vi "SDSU_ExtractInfo.vi"(8 "error in (no error)":errorcluster, 11 "refnum":i32) -> (0 "error out":errorcluster, 1 "ControllerConfigCluster":T1, 2 "Detector Type":string, 3 "refnum out":i32, 9 "PCI Info":u32[](array[numeric]) format="%.0x", 10 "Config Word Read":u32 format="%.0x")   [LabVIEW 2016]
uses:
  SDSU_GBLVariables.vi
panel:
  in  "get pci info?":bool
  in  "Default type is no info":string="optical"
  in  "Constants":i32(listbox)=5
  in  "Masks":i32(listbox)
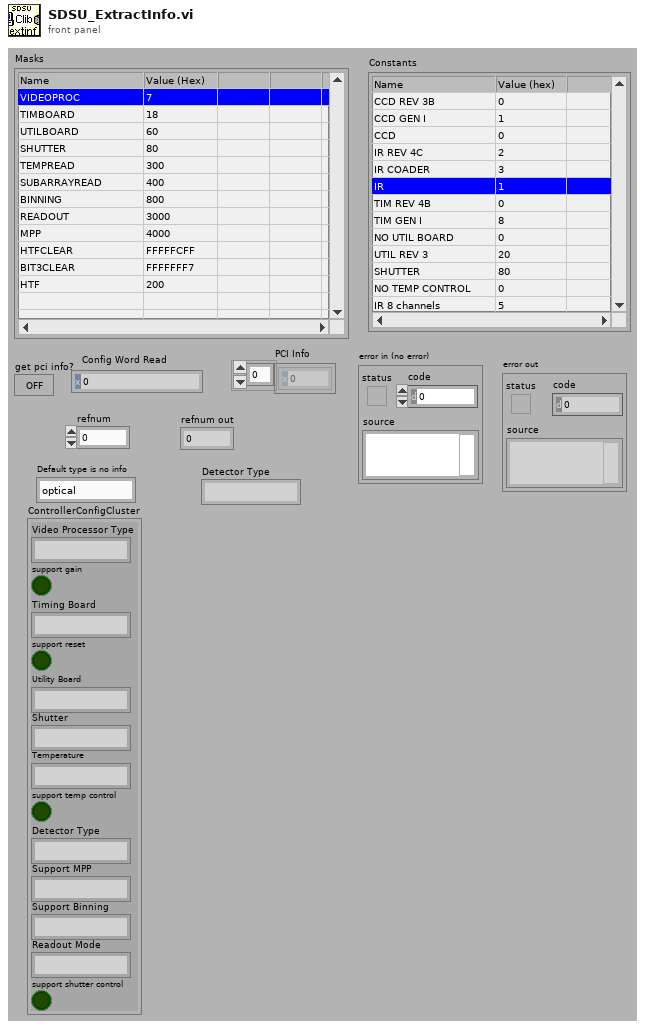
[diagram p1: front panel]
types:
  T1 = cluster{"Video Processor Type":string, "support gain":bool, "Timing Board":string, "support reset":bool, "Utility Board":string, "Shutter":string, "Temperature":string, "support temp control":bool, "Detector Type":string, "Support MPP":string, "Support Binning":string, "Readout Mode":string, "support shutter control":bool}
  T2 = cluster{"VendorID":u32, "DeviceID":u32, "RevisionNumber":u32}
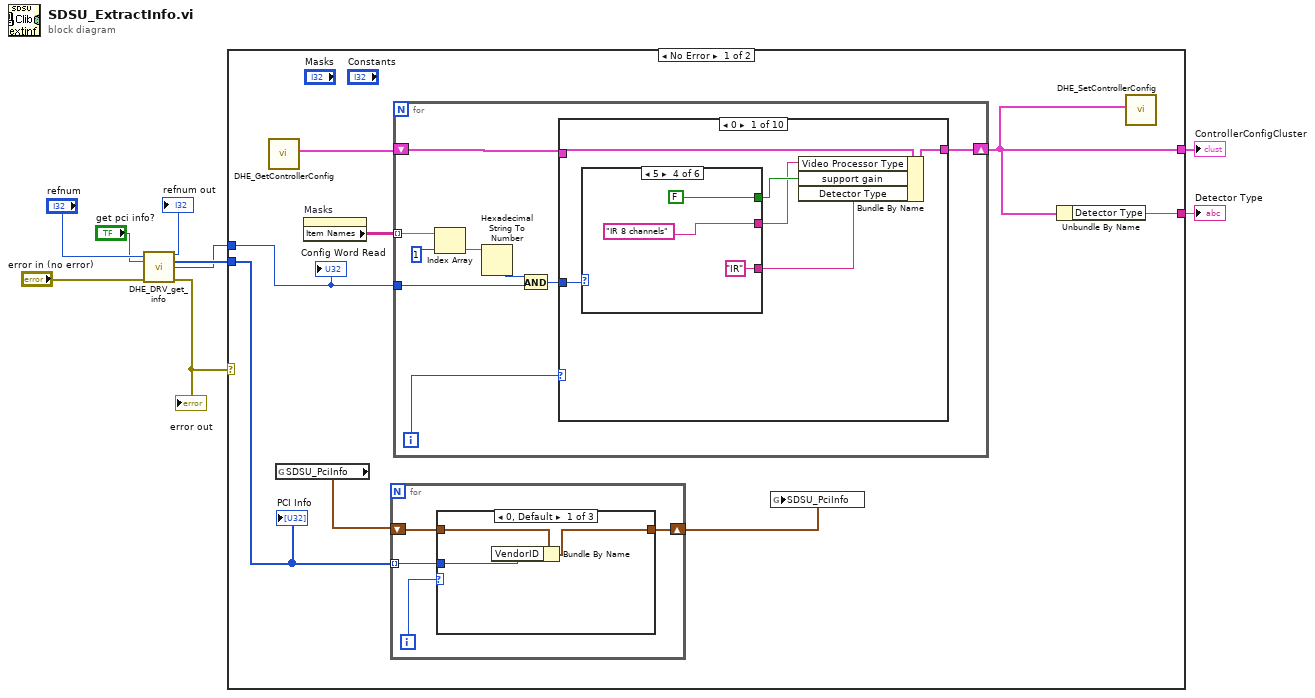
[diagram p0: block diagram]
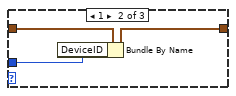
[diagram p2: hidden frame]
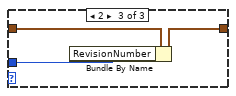
[diagram p3: hidden frame]
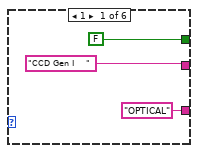
[diagram p4: hidden frame]
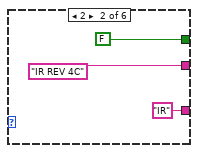
[diagram p5: hidden frame]
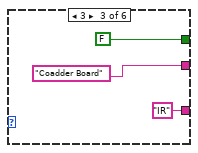
[diagram p6: hidden frame]
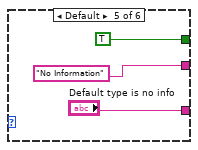
[diagram p7: hidden frame]
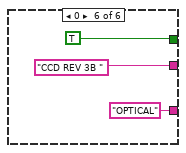
[diagram p8: hidden frame]
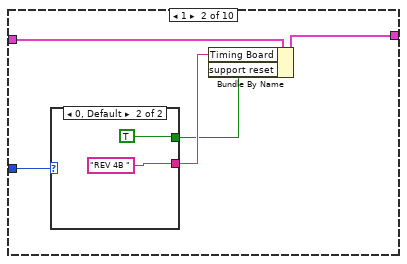
[diagram p9: hidden frame]
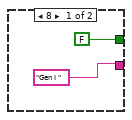
[diagram p10: hidden frame]
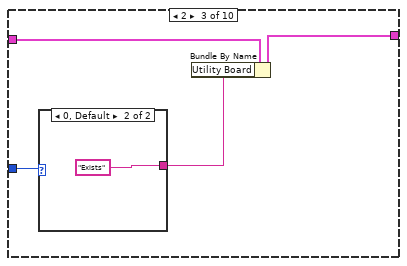
[diagram p11: hidden frame]
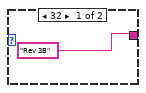
[diagram p12: hidden frame]
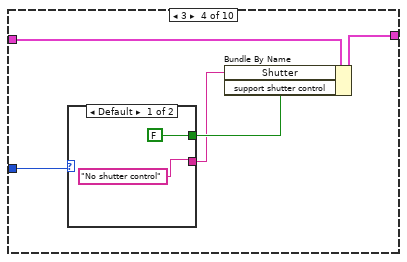
[diagram p13: hidden frame]
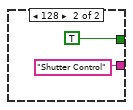
[diagram p14: hidden frame]
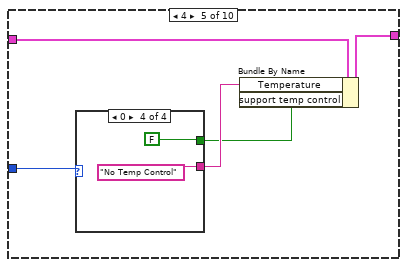
[diagram p15: hidden frame]
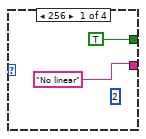
[diagram p16: hidden frame]
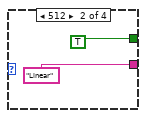
[diagram p17: hidden frame]
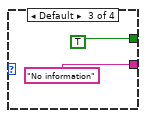
[diagram p18: hidden frame]
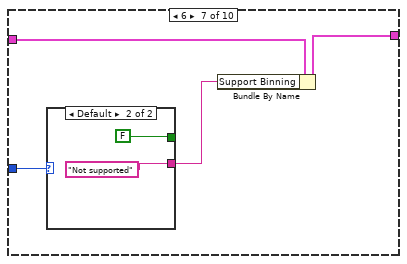
[diagram p20: hidden frame]
diagram:
  n1 = call "DHE_DRV_get_info.vi"("fd"="refnum", "get pci info?"="get pci info?", "error in (no error)"="error in (no error)") -> ("fd"=→"refnum out":i32, "Info"=w8:u16[], "error_code"=w3:i32, "error out"=w9:errorcluster)  [unwired: 9 out]
  "error out" <- w9
  n2 = case shown="No Error" w9 {
    tunnel: w3 -> [w16 _]
    tunnel: w8 -> [w15 _]
    tunnel: [w14 "UNKNOWN" ("Detector Type")] -> w6
    tunnel: [w12 T1 {"Video Processor Type"="", "support gain"=FALSE, "Timing Board"="", "support reset"=FALSE, "Utility Board"="", "Shutter"="", "Temperature"="", "support temp control"=FALSE, "Detector Type"="", "Support MPP"="", "Support Binning"="", "Readout Mode"="", "support shutter control"=FALSE} ("ControllerConfigCluster")] -> w1
    frame No Error {
      n3 = call "DHE_GetControllerConfig.vi"() -> ("ControllerConfigCluster"=w13:T1)  [unwired: 11 out]
      n4 = global read "SDSU_GBLVariables.vi" "SDSU_PciInfo"() -> (w10:T2)
      n5 = property on="Masks" class="MCListbox (strict)"() -> ("Item Names"=w17:string[][])  [unwired: 2 in, 2 out]
      n6 = for {
        tunnel: w15 -> [w19] mode=indexing
        shift-right: [w18] -> w11
        shift-left: w10 -> [w20]
        i -> [w21]
        n7 = case shown="0, Default" w21 {
          tunnel: w20 -> [w24 w27 w30]
          tunnel: w19 -> [w23 w25 w28]
          tunnel: [w22 w26 w29] -> w18
          frame 0, Default {
            n8 = Bundle By Name(cluster=w24, "VendorID"=w23) -> (w22:T2)
          }
          frame 1 {
            n9 = Bundle By Name(cluster=w27, "DeviceID"=w25) -> (w26:T2)
          }
          frame 2 {
            n10 = Bundle By Name(cluster=w30, "RevisionNumber"=w28) -> (w29:T2)
          }
        }
      }
      n11 = for {
        tunnel: w17 -> [w34] mode=indexing
        tunnel: w16 -> [w36]
        shift-right: [w31] -> w12
        shift-left: w13 -> [w32]
        i -> [w33]
        n12 = Index Array(array=w34, index=1) -> (element=w38:string)
        n13 = Hexadecimal String To Number(string=w38) -> (number=w37:u32)  [unwired: 3 out]
        n14 = And(x=w37, y=w36) -> (x .and. y?=w35:u32)
        n15 = case shown="0" w33 {
          tunnel: w35 -> [w45 w68 w76 w83 w92 _ w105 w113 w125 _]
          tunnel: w32 -> [w44 w67 w75 w82 w91 w101 w104 w112 w124 w130]
          tunnel: [w43 w66 w74 w79 w88 w101 w102 w110 w122 w130] -> w31
          frame 0 {
            n16 = case shown="5" w45 {
              tunnel: ["CCD Gen I    " "IR REV 4C" "Coadder Board" "IR 8 channels" "No Information" "CCD REV 3B "] -> w41
              tunnel: [FALSE FALSE FALSE FALSE TRUE TRUE] -> w42
              tunnel: ["OPTICAL" "IR" "IR" "IR" "Default type is no info" "OPTICAL"] -> w40
              frame 1 {
              }
              frame 2 {
              }
              frame 3 {
              }
              frame 5 {
              }
              frame Default {
              }
              frame 0 {
              }
            }
            n17 = Bundle By Name(cluster=w44, "Video Processor Type"=w41, "support gain"=w42, "Detector Type"=w40) -> (w43:T1)
          }
          frame 1 {
            n18 = case shown="0, Default" w68 {
              tunnel: ["Gen I " "REV 4B "] -> w65
              tunnel: [FALSE TRUE] -> w64
              frame 8 {
              }
              frame 0, Default {
              }
            }
            n19 = Bundle By Name(cluster=w67, "Timing Board"=w65, "support reset"=w64) -> (w66:T1)
          }
          frame 2 {
            n20 = case shown="0, Default" w76 {
              tunnel: ["Rev 3B" "Exists"] -> w73
              frame 32 {
              }
              frame 0, Default {
              }
            }
            n21 = Bundle By Name(cluster=w75, "Utility Board"=w73) -> (w74:T1)
          }
          frame 3 {
            n22 = case shown="Default" w83 {
              tunnel: ["No shutter control" "Shutter Control"] -> w80
              tunnel: [FALSE TRUE] -> w81
              frame Default {
              }
              frame 128 {
              }
            }
            n23 = Bundle By Name(cluster=w82, "Shutter"=w80, "support shutter control"=w81) -> (w79:T1)
          }
          frame 4 {
            n24 = case shown="0" w92 {
              tunnel: ["No linear" "Linear" "No information" "No Temp Control"] -> w90
              tunnel: [TRUE TRUE TRUE FALSE] -> w89
              frame 256 {
                (unwired) 2
              }
              frame 512 {
              }
              frame Default {
              }
              frame 0 {
              }
            }
            n25 = Bundle By Name(cluster=w91, "Temperature"=w90, "support temp control"=w89) -> (w88:T1)
          }
          frame 5 {
          }
          frame 6 {
            n26 = case shown="Default" w105 {
              tunnel: ["Supported" "Not supported"] -> w103
              tunnel: [TRUE FALSE] -> _
              frame 2048 {
              }
              frame Default {
              }
            }
            n27 = Bundle By Name(cluster=w104, "Support Binning"=w103) -> (w102:T1)
          }
          frame 7 {
            n28 = case shown="4096" w113 {
              tunnel: ["Lower" "Diag" "Lower and Diag" "No information"] -> w111
              tunnel: ["_CD" "_LR" "ALL" ""] -> _
              frame 4096 {
              }
              frame 8192 {
              }
              frame 12288 {
              }
              frame Default {
              }
            }
            n29 = Bundle By Name(cluster=w112, "Readout Mode"=w111) -> (w110:T1)
          }
          frame 8 {
            n30 = case shown="16384" w125 {
              tunnel: ["Supported" "No information"] -> w123
              tunnel: [TRUE FALSE] -> _
              frame 16384 {
              }
              frame Default {
              }
            }
            n31 = Bundle By Name(cluster=w124, "Support MPP"=w123) -> (w122:T1)
          }
          frame Default {
          }
        }
      }
      n32 = global write "SDSU_GBLVariables.vi" "SDSU_PciInfo"(w11) -> ()
      n33 = Unbundle By Name(w12) -> ("Detector Type"=w14:string)
      n34 = call "DHE_SetControllerConfig.vi"("ControllerConfigCluster"=w12) -> ()  [unwired: 11 out]
      "Config Word Read" <- w16
      "PCI Info" <- w15
    }
    frame Error {
    }
  }
  "Detector Type" <- w6
  "ControllerConfigCluster" <- w1
